vi "UPDATE_Export_Data_From_TXT_With_Menu_v1.1.vi"() -> ()   [LabVIEW 2018]
uses:
  <vilib>/Native 3D Graph/xcontrol/3DPC_SurfacePlot.xctl
panel:
  out "XY Graph":cluster{dbl[], dbl[]}(graph)
  out "3D Graph":refnum<class "Base Datatype.lvclass">[](xcontrol)
  out "array":dbl[][](array[numeric])
  in  "Open":bool
  in  "Выбор файла":path
  # "Z"
  # "№ отм."
  # "X"
  # "Y"
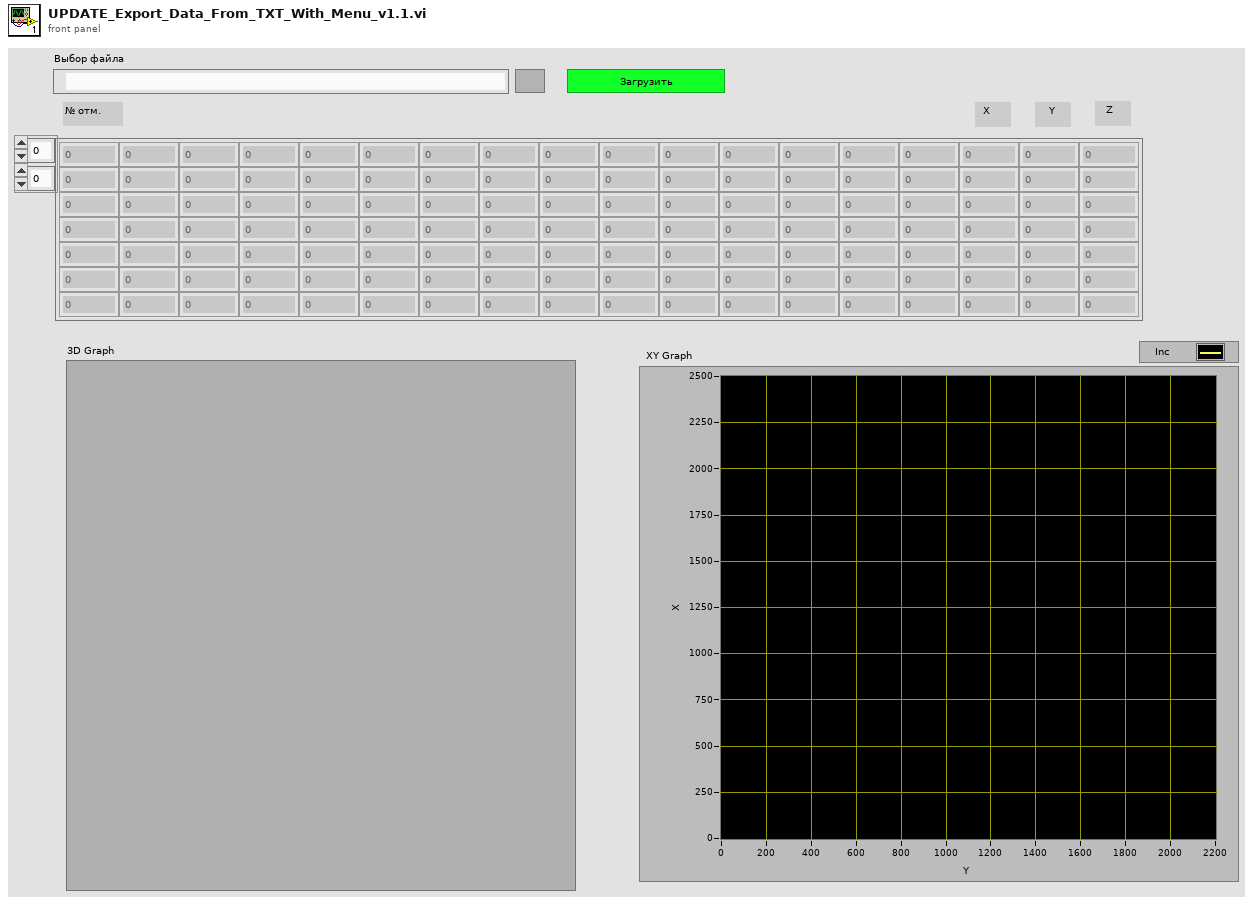
[diagram p1: front panel]
types:
  T1 = cluster{"type (empty)":dbl[], "type (empty)":dbl[]}
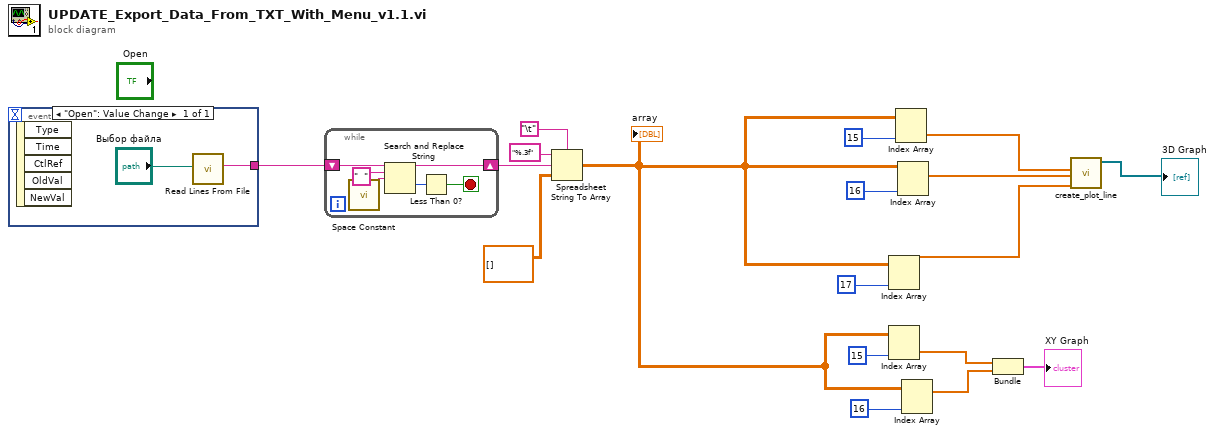
[diagram p0: block diagram]
diagram:
  n1 = event shown="[0] \"Open\": Value Change" {
    selector: _ -> [_]
    dyn-events: _ -> [_]
    timeout: _ -> [_]
    tunnel: [w20] -> w14
    event "Open": Value Change {
      n2 = event-data() -> ()  [unwired: 1 in, 5 out]
      n3 = call <vilib>:"Read Lines From File.vi"("file path (dialog if empty)"="Выбор файла") -> ("line string"=w20:string)  [unwired: 1 in, 7 out]
    }
  }
  n4 = while {
    shift-right: [w23] -> w16
    shift-left: w14 -> [w26]
    stop <- w21 stop-if-true
    n5 = call <vilib>:"Space Constant.vi"() -> ("String"=w24:string)
    n6 = Search and Replace String(input string=w26, search string="  ", replace string=w24) -> (result string=w23:string, offset past replacement=w22:i32)  [unwired: 1 in, 6 out]
    n7 = Less Than 0?(x=w22) -> (x < 0?=w21:bool)
  }
  n8 = Spreadsheet String To Array(delimiter (Tab)="\t", format string="%.3f" ("format (%.3f)"), spreadsheet string=w16, array type (2D Dbl)=dbl[][] [] ("type (empty)")) -> (array=w1:dbl[][])
  "array" <- w1
  n9 = Index Array(array=w1, index (col)=17) -> (element=w9:dbl[])  [unwired: 1 in]
  n10 = Index Array(array=w1, index (col)=15) -> (element=w3:dbl[])  [unwired: 1 in]
  n11 = Index Array(array=w1, index (col)=15) -> (element=w7:dbl[])  [unwired: 1 in]
  n12 = Index Array(array=w1, index (col)=16) -> (element=w8:dbl[])  [unwired: 1 in]
  n13 = Index Array(array=w1, index (col)=16) -> (element=w4:dbl[])  [unwired: 1 in]
  n14 = Bundle("type (empty)"=w3, "type (empty)"=w4) -> (→"XY Graph":T1)  [unwired: 1 in]
  n15 = call <vilib>:"create_plot_line.vi"("z vector"=w9, "y vector"=w8, "x vector"=w7) -> ("plots out"=→"3D Graph":refnum<class "Base Datatype.lvclass">[])  [unwired: 2 in, 6 out]
